vi "WriteSignalLog.vi"(9 "TSRefShot":bool, 10 "Ctrl_Signal":T1, 11 "refnum In":refnum<file>) -> (3 "refnum out":refnum<file>)   [LabVIEW 2016]
uses:
  Ctrl_Signal.ctl
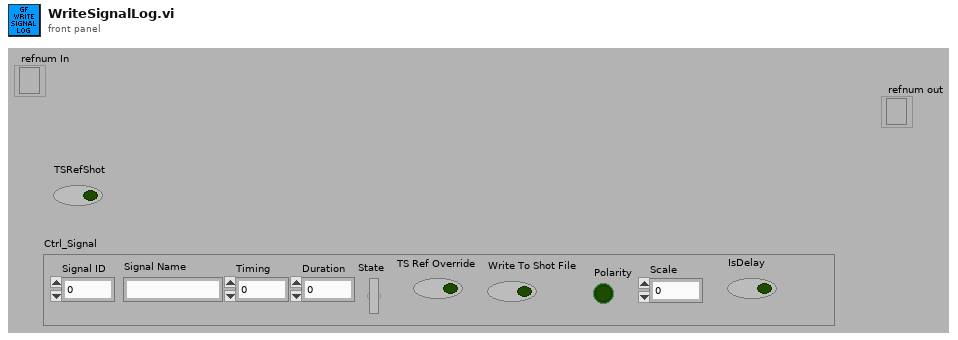
[diagram p1: front panel]
types:
  T1 = typedef "Ctrl_Signal.ctl" = cluster{"Signal Name":string, "Timing":dbl, "Duration":dbl, "State":bool, "TS Ref Override":bool, "Write To Shot File":bool, "Polarity":bool, "Signal ID":dbl, "Scale":dbl, "IsDelay":bool}
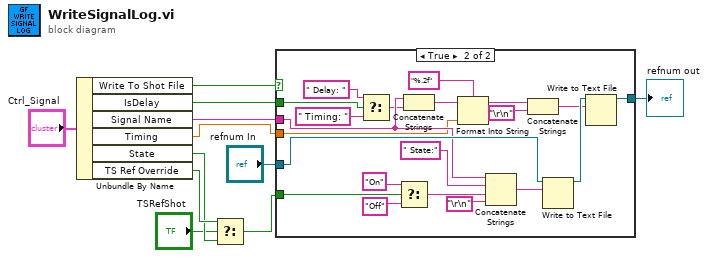
[diagram p0: block diagram]
diagram:
  n1 = Unbundle By Name("Ctrl_Signal") -> ("Write To Shot File"=w10:bool, "IsDelay"=w5:bool, "Signal Name"=w7:string, "Timing"=w6:dbl, "State"=w3:bool, "TS Ref Override"=w4:bool)
  n2 = Select(t=w4, s="TSRefShot", f=w3) -> (s? t:f=w2:bool)
  n3 = case shown="True" w10 {
    tunnel: "refnum In" -> [w12 w33]
    tunnel: [w12 w31] -> w8
    tunnel: w7 -> [_ w23]
    tunnel: w2 -> [_ w27]
    tunnel: w6 -> [_ w17]
    tunnel: w5 -> [_ w13]
    frame False {
    }
    frame True {
      n4 = Select(t=" Delay: " ("string"), s=w13, f=" Timing: " ("string")) -> (s? t:f=w16:string)
      n5 = Select(t="On" ("string"), s=w27, f="Off" ("string")) -> (s? t:f=w28:string)
      n6 = Concatenate Strings(w23, w16) -> (w22:string)
      n7 = Format Into String(format string="%.2f", initial string=w22, w17) -> (resulting string=w20:string)  [unwired: 1 in, 1 out]
      n8 = Concatenate Strings(w23, " State:" ("string"), w28, "\r\n") -> (w24:string)
      n9 = Concatenate Strings(w20, "\r\n") -> (w19:string)
      n10 = Write to Text File(file (use dialog)=w33, text=w24) -> (refnum out=w32:refnum<file>)  [unwired: 2 in, 2 out]
      n11 = Write to Text File(file (use dialog)=w32, text=w19) -> (refnum out=w31:refnum<file>)  [unwired: 2 in, 2 out]
    }
  }
  "refnum out" <- w8
